vi "Utility Decode ID String.vi"(8 "error in (no error)":errorcluster, 10 "*IDN? Response":string, 11 "VISA resource name in":refnum<visa-resource-name>) -> (0 "error out":errorcluster, 2 "Unit Info":T1, 3 "VISA resource name out":refnum<visa-resource-name>)   [LabVIEW 2012, in "Quantum Composers 9000 Series.lvlib"]
doc: "This VI decodes the response from an *IDN? query to return information about the unit It is private in scope."
uses:
  Quantum Composers 9000 Series.lvlib
  Unit Info.ctl
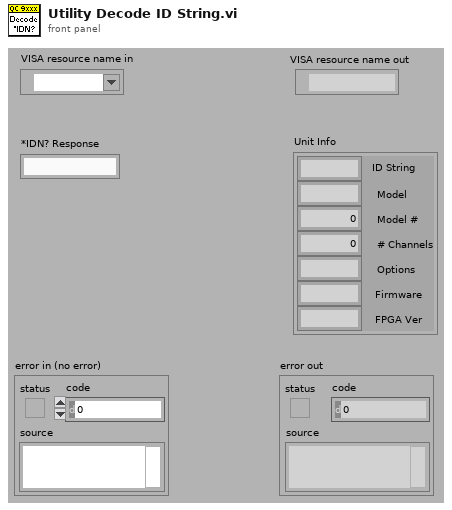
[diagram p1: front panel]
types:
  T1 = typedef "Quantum Composers 9000 Series.lvlib/Unit Info.ctl" = cluster{"ID String":string, "Model":string, "Model #":i32, "# Channels":i32, "Options":string, "Firmware":string, "FPGA Ver":string}
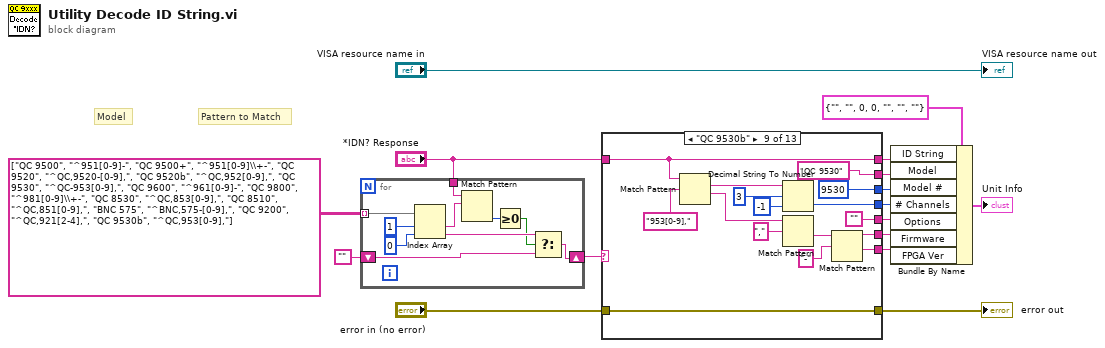
[diagram p0: block diagram]
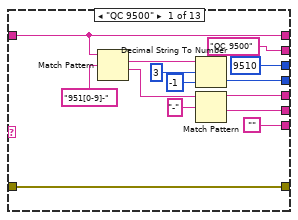
[diagram p2: hidden frame]
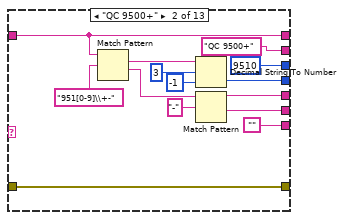
[diagram p3: hidden frame]
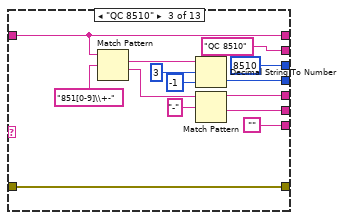
[diagram p4: hidden frame]
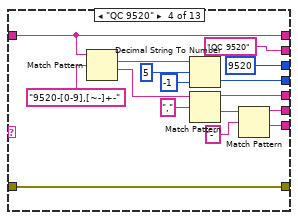
[diagram p5: hidden frame]
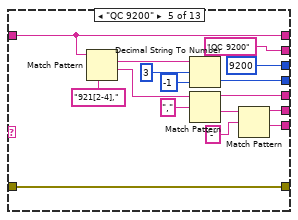
[diagram p6: hidden frame]
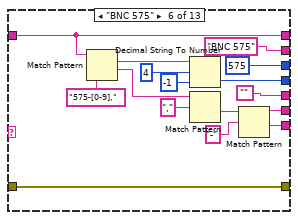
[diagram p7: hidden frame]
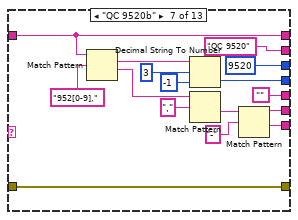
[diagram p8: hidden frame]
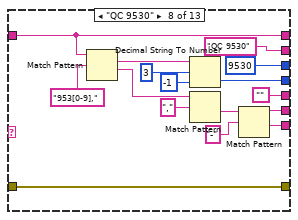
[diagram p9: hidden frame]
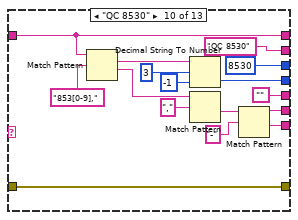
[diagram p10: hidden frame]
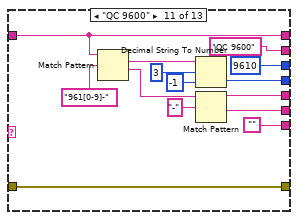
[diagram p11: hidden frame]
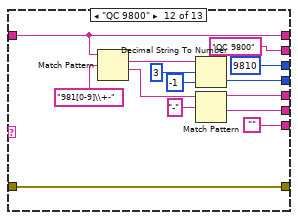
[diagram p12: hidden frame]
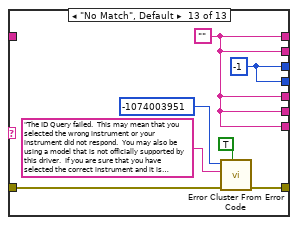
[diagram p13: hidden frame]
diagram:
  # "Pattern to Match"
  # "Model"
  n1 = for {
    tunnel: string[][] [["QC 9500", "^951[0-9]-"], ["QC 9500+", "^951[0-9]\\+-"], ["QC 9520", "^QC,9520-[0-9],"], ["QC 9520b", "^QC,952[0-9],"], ["QC 9530", "^QC-953[0-9],"], ["QC 9600", "^961[0-9]-"], ["QC 9800", "^981[0-9]\\+-"], ["QC 8530", "^QC,853[0-9],"], ["QC 8510", "^QC,851[0-9],"], ["BNC 575", "^BNC,575-[0-9],"], ["QC 9200", "^QC,921[2-4],"], ["QC 9530b", "^QC,953[0-9],"]] ("appended array") -> [w24] mode=indexing
    tunnel: "*IDN? Response" -> [w25]
    shift-right: [w18] -> w6
    shift-left: "" -> [w19]
    n2 = Index Array(array=w24, index #1=1 ("index"), index #2=0 ("index")) -> (element #1=w23:string, element #2=w20:string)
    n3 = Match Pattern(string=w25, regular expression=w23) -> (offset past match=w26:i32)  [unwired: 4 out]
    n4 = Greater Or Equal To 0?(x=w26) -> (x >= 0?=w17:bool)
    n5 = Select(t=w20, s=w17, f=w19) -> (s? t:f=w18:string)
  }
  n6 = case shown="\"QC 9530b\"" w6 {
    tunnel: "*IDN? Response" -> [w38 w52 w66 w82 w98 w114 w130 w146 w162 w178 w192 w206 _]
    tunnel: [w38 w52 w66 w82 w98 w114 w130 w146 w162 w178 w192 w206 w214] -> w7
    tunnel: ["QC 9500" ("Model") "QC 9500+" ("Model") "QC 8510" ("Model") "QC 9520" ("Model") "QC 9200" ("Model") "BNC 575" ("Model") "QC 9520" ("Model") "QC 9530" ("Model") "QC 9530" ("Model") "QC 8530" ("Model") "QC 9600" ("Model") "QC 9800" ("Model") w214] -> w8
    tunnel: [9510 ("Model #") 9510 ("Model #") 8510 ("Model #") 9520 ("Model #") 9200 ("Model #") 575 ("Model #") 9520 ("Model #") 9530 ("Model #") 9530 ("Model #") 8530 ("Model #") 9610 ("Model #") 9810 ("Model #") w215] -> w9
    tunnel: [w35 w49 w63 w79 w95 w111 w127 w143 w159 w175 w189 w203 w215] -> w10
    tunnel: [w31 w45 w59 w77 w93 "" "" "" "" "" w185 w199 w214] -> w11
    tunnel: [w30 w44 w58 w72 w88 w105 w121 w137 w153 w169 w184 w198 w214] -> w12
    tunnel: ["" "" "" w71 w87 w104 w120 w136 w152 w168 "" "" w214] -> w13
    tunnel: "error in (no error)" -> [w27 w41 w55 w69 w85 w102 w118 w134 w150 w166 w181 w195 w210]
    tunnel: [w27 w41 w55 w69 w85 w102 w118 w134 w150 w166 w181 w195 w209] -> w4
    frame "QC 9500" {
      n7 = Match Pattern(string=w38, regular expression="951[0-9]-") -> (match substring=w34:string, after substring=w32:string)  [unwired: 3 out]
      n8 = Decimal String To Number(string=w34, offset=3, default (0L)=-1) -> (number=w35:i32)  [unwired: 1 out]
      n9 = Match Pattern(string=w32, regular expression="-") -> (before substring=w31:string, after substring=w30:string)  [unwired: 3 out]
    }
    frame "QC 9500+" {
      n10 = Match Pattern(string=w52, regular expression="951[0-9]\\+-") -> (match substring=w48:string, after substring=w46:string)  [unwired: 3 out]
      n11 = Decimal String To Number(string=w48, offset=3, default (0L)=-1) -> (number=w49:i32)  [unwired: 1 out]
      n12 = Match Pattern(string=w46, regular expression="-") -> (before substring=w45:string, after substring=w44:string)  [unwired: 3 out]
    }
    frame "QC 8510" {
      n13 = Match Pattern(string=w66, regular expression="851[0-9]\\+-") -> (match substring=w62:string, after substring=w60:string)  [unwired: 3 out]
      n14 = Decimal String To Number(string=w62, offset=3, default (0L)=-1) -> (number=w63:i32)  [unwired: 1 out]
      n15 = Match Pattern(string=w60, regular expression="-") -> (before substring=w59:string, after substring=w58:string)  [unwired: 3 out]
    }
    frame "QC 9520" {
      n16 = Match Pattern(string=w82, regular expression="9520-[0-9],[~-]+-") -> (match substring=w76:string, after substring=w75:string)  [unwired: 3 out]
      n17 = Decimal String To Number(string=w76, offset=5, default (0L)=-1) -> (number=w79:i32)  [unwired: 1 out]
      n18 = Match Pattern(string=w75, regular expression=",") -> (before substring=w77:string, after substring=w73:string)  [unwired: 3 out]
      n19 = Match Pattern(string=w73, regular expression="-") -> (before substring=w72:string, after substring=w71:string)  [unwired: 3 out]
    }
    frame "QC 9200" {
      n20 = Match Pattern(string=w98, regular expression="921[2-4],") -> (match substring=w92:string, after substring=w91:string)  [unwired: 3 out]
      n21 = Decimal String To Number(string=w92, offset=3, default (0L)=-1) -> (number=w95:i32)  [unwired: 1 out]
      n22 = Match Pattern(string=w91, regular expression=",") -> (before substring=w93:string, after substring=w89:string)  [unwired: 3 out]
      n23 = Match Pattern(string=w89, regular expression="-") -> (before substring=w88:string, after substring=w87:string)  [unwired: 3 out]
    }
    frame "BNC 575" {
      n24 = Match Pattern(string=w114, regular expression="575-[0-9],") -> (match substring=w109:string, after substring=w108:string)  [unwired: 3 out]
      n25 = Decimal String To Number(string=w109, offset=4, default (0L)=-1) -> (number=w111:i32)  [unwired: 1 out]
      n26 = Match Pattern(string=w108, regular expression=",") -> (after substring=w106:string)  [unwired: 4 out]
      n27 = Match Pattern(string=w106, regular expression="-") -> (before substring=w105:string, after substring=w104:string)  [unwired: 3 out]
    }
    frame "QC 9520b" {
      n28 = Match Pattern(string=w130, regular expression="952[0-9],") -> (match substring=w125:string, after substring=w124:string)  [unwired: 3 out]
      n29 = Decimal String To Number(string=w125, offset=3, default (0L)=-1) -> (number=w127:i32)  [unwired: 1 out]
      n30 = Match Pattern(string=w124, regular expression=",") -> (after substring=w122:string)  [unwired: 4 out]
      n31 = Match Pattern(string=w122, regular expression="-") -> (before substring=w121:string, after substring=w120:string)  [unwired: 3 out]
    }
    frame "QC 9530" {
      n32 = Match Pattern(string=w146, regular expression="953[0-9],") -> (match substring=w141:string, after substring=w140:string)  [unwired: 3 out]
      n33 = Decimal String To Number(string=w141, offset=3, default (0L)=-1) -> (number=w143:i32)  [unwired: 1 out]
      n34 = Match Pattern(string=w140, regular expression=",") -> (after substring=w138:string)  [unwired: 4 out]
      n35 = Match Pattern(string=w138, regular expression="-") -> (before substring=w137:string, after substring=w136:string)  [unwired: 3 out]
    }
    frame "QC 9530b" {
      n36 = Match Pattern(string=w162, regular expression="953[0-9],") -> (match substring=w157:string, after substring=w156:string)  [unwired: 3 out]
      n37 = Decimal String To Number(string=w157, offset=3, default (0L)=-1) -> (number=w159:i32)  [unwired: 1 out]
      n38 = Match Pattern(string=w156, regular expression=",") -> (after substring=w154:string)  [unwired: 4 out]
      n39 = Match Pattern(string=w154, regular expression="-") -> (before substring=w153:string, after substring=w152:string)  [unwired: 3 out]
    }
    frame "QC 8530" {
      n40 = Match Pattern(string=w178, regular expression="853[0-9],") -> (match substring=w173:string, after substring=w172:string)  [unwired: 3 out]
      n41 = Decimal String To Number(string=w173, offset=3, default (0L)=-1) -> (number=w175:i32)  [unwired: 1 out]
      n42 = Match Pattern(string=w172, regular expression=",") -> (after substring=w170:string)  [unwired: 4 out]
      n43 = Match Pattern(string=w170, regular expression="-") -> (before substring=w169:string, after substring=w168:string)  [unwired: 3 out]
    }
    frame "QC 9600" {
      n44 = Match Pattern(string=w192, regular expression="961[0-9]-") -> (match substring=w188:string, after substring=w186:string)  [unwired: 3 out]
      n45 = Decimal String To Number(string=w188, offset=3, default (0L)=-1) -> (number=w189:i32)  [unwired: 1 out]
      n46 = Match Pattern(string=w186, regular expression="-") -> (before substring=w185:string, after substring=w184:string)  [unwired: 3 out]
    }
    frame "QC 9800" {
      n47 = Match Pattern(string=w206, regular expression="981[0-9]\\+-") -> (match substring=w202:string, after substring=w200:string)  [unwired: 3 out]
      n48 = Decimal String To Number(string=w202, offset=3, default (0L)=-1) -> (number=w203:i32)  [unwired: 1 out]
      n49 = Match Pattern(string=w200, regular expression="-") -> (before substring=w199:string, after substring=w198:string)  [unwired: 3 out]
    }
    frame "No Match", Default {
      w215 = -1 ("Model #")
      w214 = ""
      n50 = call <vilib>:"Error Cluster From Error Code.vi"("show call chain? (False)"=TRUE, "error in (no error)"=w210, "error message (\"\")"="The ID Query failed.  This may mean that you selected the wrong instrument or your instrument did not respond.  You may also be using a model that is not officially supported by this driver.  If you are sure that you have selected the correct instrument and it is responding, try disabling the ID Query." ("Source (VI Name)"), "error code (0)"=-1074003951 ("Code")) -> ("error out"=w209:errorcluster)  [unwired: 5 out]
    }
  }
  "error out" <- w4
  n51 = Bundle By Name(cluster=T1 {"ID String"="", "Model"="", "Model #"=0, "# Channels"=0, "Options"="", "Firmware"="", "FPGA Ver"=""} ("Unit Info"), "ID String"=w7, "Model"=w8, "Model #"=w9, "# Channels"=w10, "Options"=w11, "Firmware"=w12, "FPGA Ver"=w13) -> (→"Unit Info":T1)
  "VISA resource name out" <- "VISA resource name in"
